vi "parfor_progress.vi"(7 "Parpool Count":i32, 8 "Current Display":i32, 9 "PID":i32, 10 "reset":bool, 11 "N":i32) -> (0 "Processing Rate":dbl, 1 "Display Array":i32[](array[numeric]), 3 "Percent Count":i32)   [LabVIEW 2019]
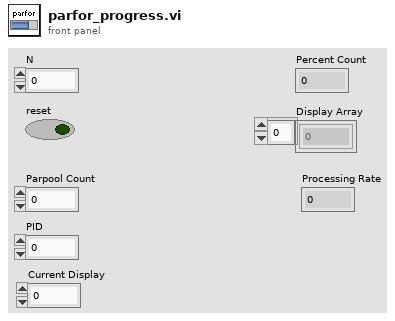
[diagram p1: front panel]
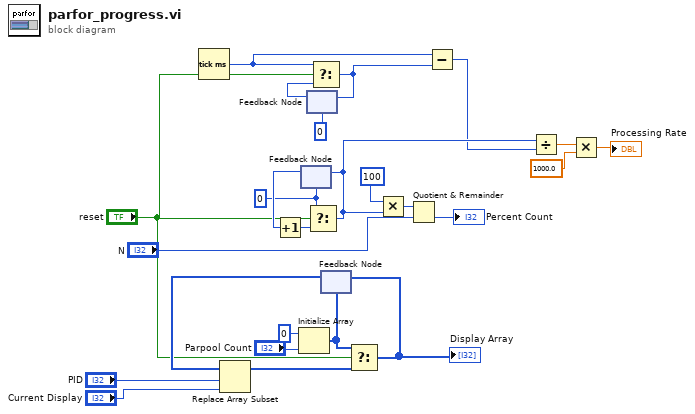
[diagram p0: block diagram]
diagram:
  w24 = 0
  n1 = Tick Count (ms)() -> (millisecond timer value=w6:u32)
  n2 = Initialize Array(0 ("element"), "Parpool Count") -> (w15:i32[])
  n3 = feedback #1(w24) -> (w25:i32)
  n4 = Increment(x=w25) -> (x+1=w23:i32)
  n5 = feedback #2(u32 0 ("millisecond timer value")) -> (w9:u32)
  n6 = Select(t=w24, s="reset", f=w23) -> (s? t:f=w5:i32)
  n7 = feedback-in #1(w5) -> ()
  n8 = Select(t=w6, s="reset", f=w9) -> (s? t:f=w7:u32)
  n9 = feedback-in #2(w7) -> ()
  n10 = feedback #3(w15) -> (w14:i32[])
  n11 = Replace Array Subset(array=w14, new element="Current Display", index="PID") -> (w11:i32[])
  n12 = Select(t=w15, s="reset", f=w11) -> (s? t:f=w18:i32[])
  "Display Array" <- w18
  n13 = feedback-in #3(w18) -> ()
  n14 = Multiply(x=100, y=w5) -> (x*y=w22:i32)
  n15 = Quotient & Remainder(x=w22, y="N") -> (floor(x/y)=→"Percent Count":i32)  [unwired: 1 out]
  n16 = Subtract(x=w6, y=w7) -> (x-y=w4:u32)
  n17 = Divide(x=w5, y=w4) -> (x/y=w3:dbl)
  n18 = Multiply(x=w3, y=1000.0) -> (x*y=→"Processing Rate":dbl)
